vi "fmt_formatColumnHeaders.vi"(8 "error in":errorcluster, 11 "column headers":string[](array[string])) -> (0 "error out":errorcluster, 3 "formatted column headers":string)   [LabVIEW 2020, in "NI_ExcelFile.lvlib"]
uses:
  <vilib>/express/express shared/NI_ExcelFile/NI_ExcelFile.lvlib
  <vilib>/express/express shared/NI_ExcelFile/SubVIs/fmt_getUTF-8Text.vi
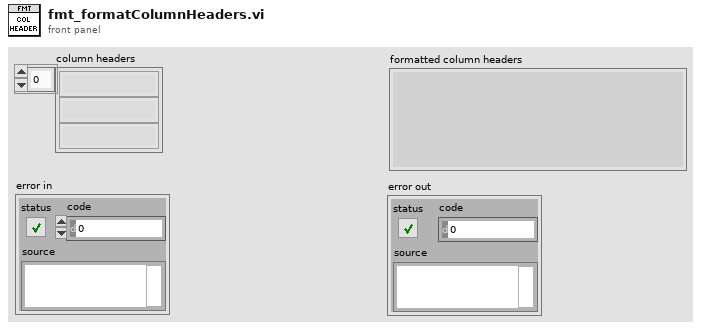
[diagram p1: front panel]
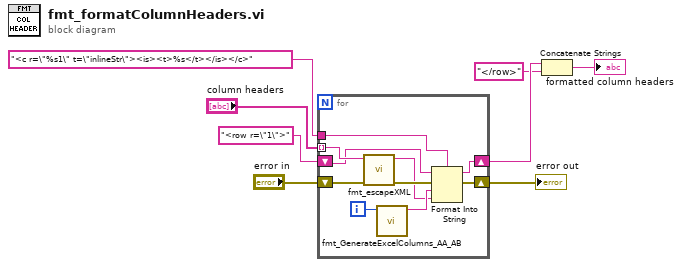
[diagram p0: block diagram]
diagram:
  n1 = for {
    tunnel: "column headers" -> [w18] mode=indexing
    tunnel: "<c r=\"%s1\" t=\"inlineStr\"><is><t>%s</t></is></c>" -> [w16]
    shift-right: [w13] -> w3
    shift-left: "<row r=\"1\">" -> [w17]
    shift-right: [w12] -> w6
    shift-left: "error in" -> [w11]
    i -> [w15]
    n2 = call <vilib>:"fmt_escapeXML.vi"("error in"=w11, "plain text"=w18) -> ("error out"=w10:errorcluster, "xml text"=w9:string)  [unwired: 8 in]
    n3 = call <vilib>:"fmt_GenerateExcelColumns_AA_AB.vi"("NumColumns"=w15) -> ("Column"=w14:string)  [unwired: 10 in]
    n4 = Format Into String(format string=w16, initial string=w17, error in=w10, w14, w9) -> (resulting string=w13:string, error out=w12:errorcluster)
  }
  "error out" <- w6
  n5 = Concatenate Strings(w3, "</row>" ("string")) -> (→"formatted column headers":string)
